vi "evaluate_expression.vi"(8 "error in (no error)":errorcluster, 10 "values":dbl[](array[numeric]), 11 "expression":string) -> (0 "error out":errorcluster, 2 "result":dbl)   [LabVIEW 2010]
doc: "Use this template to build a VI to use as a subVI."
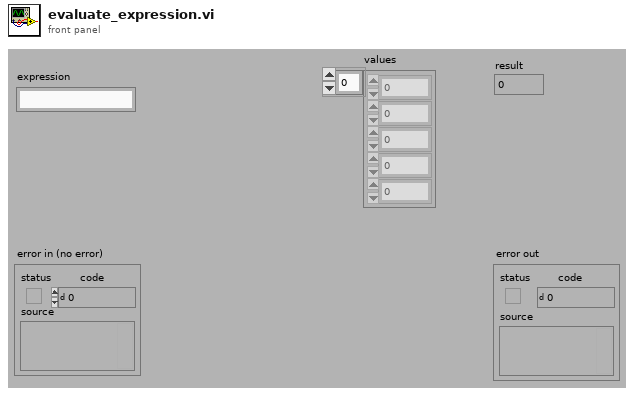
[diagram p1: front panel]
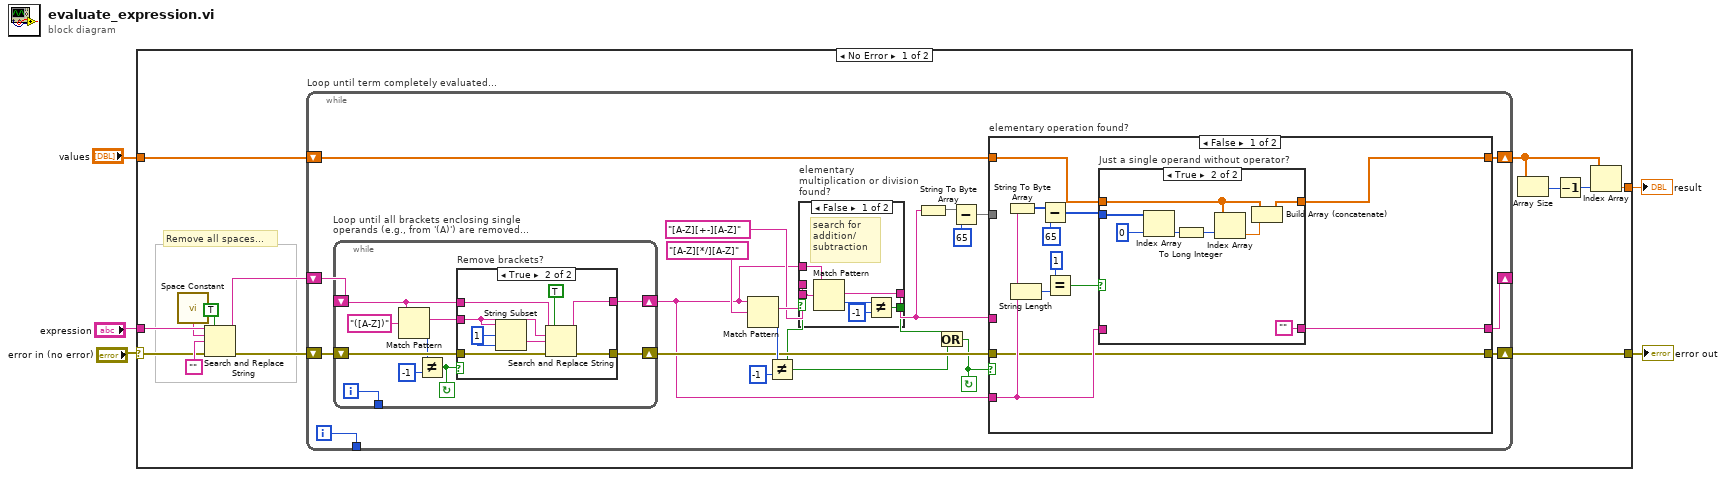
[diagram p0: block diagram]
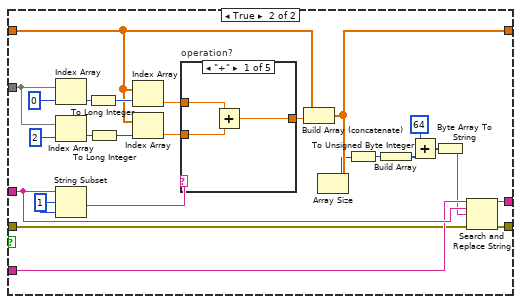
[diagram p4: hidden frame]
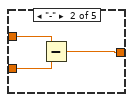
[diagram p5: hidden frame]
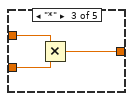
[diagram p6: hidden frame]
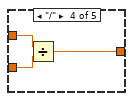
[diagram p7: hidden frame]
diagram:
  n1 = case shown="No Error" "error in (no error)" {
    selector: "error in (no error)" -> [w11 w125]
    tunnel: [w10 w125] -> w2
    tunnel: "expression" -> [w18 _]
    tunnel: "values" -> [w12 _]
    tunnel: [w8 _] -> w1
    frame No Error {
      # "Remove all spaces..."
      n2 = call <vilib>:"Space Constant.vi"() -> ("String"=w17:string)
      n3 = Search and Replace String(replace all?=TRUE ("replace all? (F)"), input string=w18, search string=w17, replace string="", error in=w11) -> (result string=w13:string, error out=w14:errorcluster)  [unwired: 5 out]
      n4 = while "Loop until term completely evaluated..." {
        shift-right: [w31] -> w9
        shift-left: w12 -> [w32]
        shift-right: [w33] -> w10
        shift-left: w14 -> [w38]
        shift-right: [w20] -> _
        shift-left: w13 -> [w37]
        tunnel: [w19] -> _
        i -> [w19]
        stop <- w21 continue-if-true
        n5 = while "Loop until all brackets enclosing single operands (e.g., from '(A)') are removed..." {
          shift-right: [w112] -> w34
          shift-left: w38 -> [w113]
          shift-right: [w111] -> w24
          shift-left: w37 -> [w106]
          tunnel: [w105] -> _
          i -> [w105]
          stop <- w107 continue-if-true
          n6 = Match Pattern(string=w106, regular expression="([A-Z])") -> (match substring=w110:string, offset past match=w109:i32)  [unwired: 3 out]
          n7 = Not Equal?(x=w109, y=-1) -> (x != y?=w107:bool)
          n8 = case "Remove brackets?" shown="True" w107 {
            tunnel: w113 -> [w115 w124]
            tunnel: [w115 w123] -> w112
            tunnel: w106 -> [w116 w121]
            tunnel: [w116 w120] -> w111
            tunnel: w110 -> [_ w118]
            frame False {
            }
            frame True {
              w119 = 1 ("offset (0)")
              n9 = String Subset(string=w118, offset (0)=w119, length (rest)=w119) -> (substring=w117:string)
              n10 = Search and Replace String(replace all?=TRUE ("replace all? (F)"), input string=w121, search string=w118, replace string=w117, error in=w124) -> (result string=w120:string, error out=w123:errorcluster)  [unwired: 5 out]
            }
          }
        }
        n11 = Match Pattern(string=w24, regular expression="[A-Z][*/][A-Z]") -> (match substring=w27:string, offset past match=w35:i32)  [unwired: 3 out]
        n12 = Not Equal?(x=w35, y=-1) -> (x != y?=w22:bool)
        n13 = case "elementary multiplication or division found?" shown="False" w22 {
          tunnel: w27 -> [_ w46]
          tunnel: [w45 w46] -> w26
          tunnel: "[A-Z][+-][A-Z]" ("regular expression") -> [w44 _]
          tunnel: w24 -> [w43 _]
          tunnel: [w40 _] -> w23
          frame False {
            # "search for addition/subtraction"
            n14 = Match Pattern(string=w43, regular expression=w44) -> (match substring=w45:string, offset past match=w41:i32)  [unwired: 3 out]
            n15 = Not Equal?(x=w41, y=-1) -> (x != y?=w40:bool)
          }
          frame True {
          }
        }
        n16 = String To Byte Array(string=w26) -> (unsigned byte array=w30:u8[])
        n17 = Or(x=w23, y=w22) -> (x .or. y?=w21:bool)
        n18 = Subtract(x=w30, y=u8 65) -> (x-y=w29:u8[])
        n19 = case "elementary operation found?" shown="False" w21 {
          tunnel: w34 -> [w48 w68]
          tunnel: [w48 w81] -> w33
          tunnel: w32 -> [w54 w82]
          tunnel: [w53 w77] -> w31
          tunnel: w29 -> [_ w91]
          tunnel: w26 -> [_ w80]
          tunnel: w24 -> [w49 w79]
          tunnel: [w47 w78] -> w20
          frame False {
            n20 = String To Byte Array(string=w49) -> (unsigned byte array=w52:u8[])
            n21 = String Length(string=w49) -> (length=w57:i32)
            n22 = Subtract(x=w52, y=u8 65) -> (x-y=w50:u8[])
            n23 = Equal?(x=1, y=w57) -> (x = y?=w55:bool)
            n24 = case "Just a single operand without operator?" shown="True" w55 {
              tunnel: w50 -> [_ w64]
              tunnel: w54 -> [w59 w62]
              tunnel: [w59 w61] -> w53
              tunnel: w49 -> [w58 _]
              tunnel: [w58 ""] -> w47
              frame False {
              }
              frame True {
                n25 = Index Array(array=w64, index=0 ("offset (0)")) -> (element=w66:u8)
                n26 = To Long Integer(number=w66) -> (32bit integer=w65:i32)
                n27 = Index Array(array=w62, index=w65) -> (element=w63:dbl)
                n28 = Build Array (concatenate)(w62, w63) -> (w61:dbl[])
              }
            }
          }
          frame True {
            w89 = 1 ("offset (0)")
            n29 = Index Array(array=w91, index=0 ("offset (0)")) -> (element=w87:u8)
            n30 = Index Array(array=w91, index=2 ("offset (0)")) -> (element=w85:u8)
            n31 = String Subset(string=w80, offset (0)=w89, length (rest)=w89) -> (substring=w88:string)
            n32 = To Long Integer(number=w87) -> (32bit integer=w86:i32)
            n33 = To Long Integer(number=w85) -> (32bit integer=w84:i32)
            n34 = Index Array(array=w82, index=w86) -> (element=w70:dbl)
            n35 = Index Array(array=w82, index=w84) -> (element=w83:dbl)
            n36 = case "operation?" shown="\"+\"" w88 {
              tunnel: w83 -> [w94 w97 w101 w103 _]
              tunnel: w70 -> [w95 w98 w100 w104 _]
              tunnel: [w93 w96 w99 w102 _] -> w69
              frame "+" {
                n37 = Add(x=w95, y=w94) -> (x+y=w93:dbl)
              }
              frame "-" {
                n38 = Subtract(x=w98, y=w97) -> (x-y=w96:dbl)
              }
              frame "*" {
                n39 = Multiply(x=w100, y=w101) -> (x*y=w99:dbl)
              }
              frame "/" {
                n40 = Divide(x=w104, y=w103) -> (x/y=w102:dbl)
              }
              frame Default {
                # "none (should not happen anyway)..."
              }
            }
            n41 = Build Array (concatenate)(w82, w69) -> (w77:dbl[])
            n42 = Array Size(array=w77) -> (size(s)=w76:i32)
            n43 = To Unsigned Byte Integer(number=w76) -> (unsigned 8bit integer=w75:u8)
            n44 = Build Array(w75) -> (w73:u8[])
            n45 = Add(x=u8 64, y=w73) -> (x+y=w72:u8[])
            n46 = Byte Array To String(unsigned byte array=w72) -> (string=w71:string)
            n47 = Search and Replace String(input string=w79, search string=w80, replace string=w71, error in=w68) -> (result string=w78:string, error out=w81:errorcluster)  [unwired: 6 out]
          }
        }
      }
      n48 = Array Size(array=w9) -> (size(s)=w7:i32)
      n49 = Decrement(x=w7) -> (x-1=w6:i32)
      n50 = Index Array(array=w9, index=w6) -> (element=w8:dbl)
    }
    frame Error {
    }
  }
  "error out" <- w2
  "result" <- w1
